vi "QueueDriver.vi"(0 "Queue Name":string, 5 "Enqueue State":string, 7 "Array State":string[](array[string]), 11 "error in":errorcluster, 13 "Queue Operations":T1) -> (4 "Dequeue State":string, 15 "error out":errorcluster)   [LabVIEW 2023]
doc: "This is the simple queue driver which can enqueue and dequeue states into a queue and use it further."
uses:
  Typedef/QueueOperations.ctl
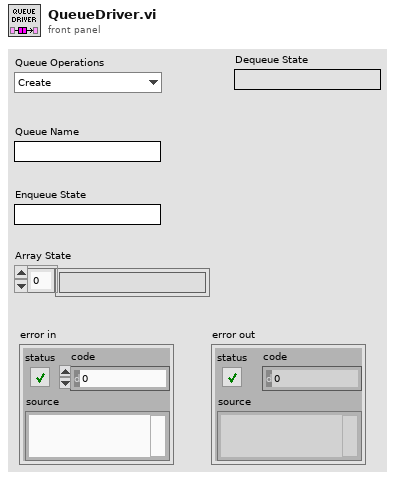
[diagram p1: front panel]
types:
  T1 = typedef "QueueOperations.ctl" = enum16{"Create", "Enqueue", "Enqueue N elements", "Dequeue", "Flush", "Release"}
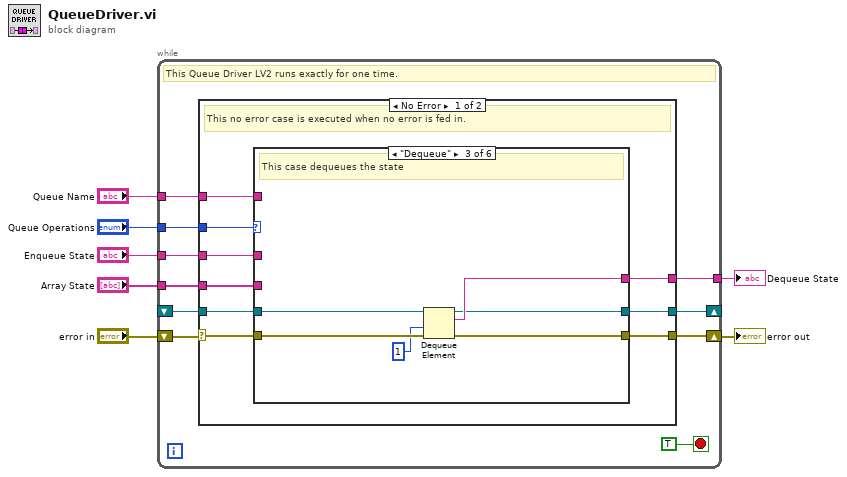
[diagram p0: block diagram]
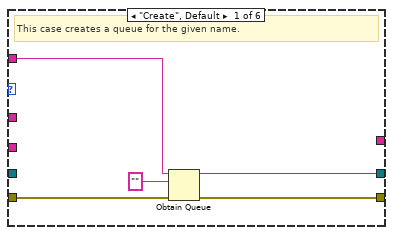
[diagram p2: hidden frame]
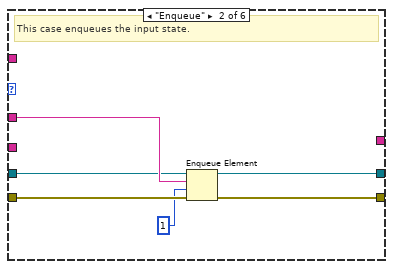
[diagram p3: hidden frame]
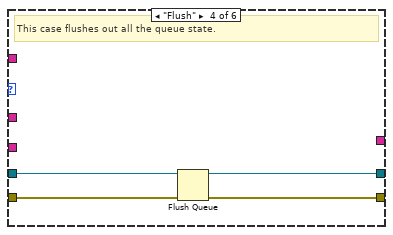
[diagram p4: hidden frame]
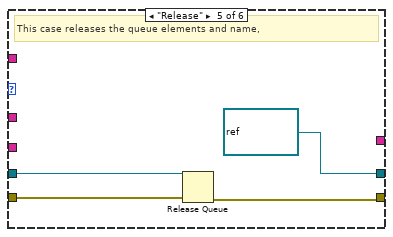
[diagram p5: hidden frame]
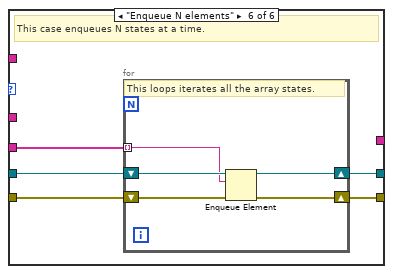
[diagram p6: hidden frame]
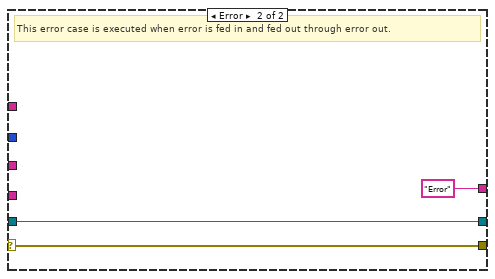
[diagram p7: hidden frame]
diagram:
  n1 = while {
    shift-right: [w15] -> w6
    shift-left: "error in" -> [w17]
    tunnel: "Queue Operations" -> [w16]
    tunnel: "Queue Name" -> [w14]
    tunnel: "Enqueue State" -> [w13]
    tunnel: [w11] -> w2
    shift-right: [w10] -> _
    shift-left: _ -> [w9]
    tunnel: "Array State" -> [w8]
    stop <- TRUE stop-if-true
    # "This Queue Driver LV2 runs exactly for one time."
    n2 = case shown="No Error" w17 {
      selector: w17 -> [w25 w64]
      tunnel: w16 -> [w26 _]
      tunnel: [w24 w64] -> w15
      tunnel: w14 -> [w23 _]
      tunnel: w13 -> [w22 _]
      tunnel: [w21 "Error" ("element")] -> w11
      tunnel: [w20 w62] -> w10
      tunnel: w9 -> [w19 w62]
      tunnel: w8 -> [w18 _]
      frame No Error {
        # "This no error case is executed when no error is fed in."
        n3 = case shown="\"Dequeue\"" w26 {
          tunnel: w25 -> [w31 w37 w43 w47 w51 w56]
          tunnel: [w30 w36 w42 w46 w50 w54] -> w24
          tunnel: w23 -> [w29 _ _ _ _ _]
          tunnel: w22 -> [_ w35 _ _ _ _]
          tunnel: [_ _ w41 _ _ _] -> w21
          tunnel: [w28 w34 w40 w45 refnum<queue> refnum ("queue out") w53] -> w20
          tunnel: w19 -> [_ w33 w39 w44 w49 w55]
          tunnel: w18 -> [_ _ _ _ _ w52]
          frame "Create", Default {
            # "This case creates a queue for the given name."
            n4 = Obtain Queue(name (unnamed)=w29, element data type="", error in (no error)=w31) -> (queue out=w28:refnum<queue>, error out=w30:errorcluster)  [unwired: 2 in, 1 out]
          }
          frame "Enqueue" {
            # "This case enqueues the input state."
            n5 = Enqueue Element(queue=w33, element=w35, timeout in ms (-1)=1, error in (no error)=w37) -> (queue out=w34:refnum<queue>, error out=w36:errorcluster)  [unwired: 1 out]
          }
          frame "Dequeue" {
            # "This case dequeues the state"
            n6 = Dequeue Element(queue=w39, timeout in ms (-1)=1, error in (no error)=w43) -> (queue out=w40:refnum<queue>, element=w41:string, error out=w42:errorcluster)  [unwired: 1 out]
          }
          frame "Flush" {
            # "This case flushes out all the queue state."
            n7 = Flush Queue(queue=w44, error in (no error)=w47) -> (queue out=w45:refnum<queue>, error out=w46:errorcluster)  [unwired: 1 out]
          }
          frame "Release" {
            # "This case releases the queue elements and name,"
            n8 = Release Queue(queue=w49, error in (no error)=w51) -> (error out=w50:errorcluster)  [unwired: 1 in, 2 out]
          }
          frame "Enqueue N elements" {
            # "This case enqueues N states at a time."
            n9 = for {
              shift-right: [w58] -> w53
              shift-left: w55 -> [w59]
              shift-right: [w60] -> w54
              shift-left: w56 -> [w61]
              tunnel: w52 -> [w57] mode=indexing
              # "This loops iterates all the array states."
              n10 = Enqueue Element(queue=w59, element=w57, error in (no error)=w61) -> (queue out=w58:refnum<queue>, error out=w60:errorcluster)  [unwired: 1 in, 1 out]
            }
          }
        }
      }
      frame Error {
        # "This error case is executed when error is fed in and fed out through error out."
      }
    }
  }
  "error out" <- w6
  "Dequeue State" <- w2
